vi "Title Font Read.vi"(4 "error in (no error)":errorcluster, 6 "Container State":T14, 7 "Display State In":T1={"Properties"={"Chart"={"ChartName"="Chart", "AntiAliasing"=3, "background"={"Color"={"Color"=0, "alpha"=76}, "HatchStyle"=76, "GradientStyle"=0}}, "ChartArea"={"Background"={"Color"={"Color"=0, "alpha"=76}, "HatchStyle"=76, "GradientStyle"=0}, "Border"={"color"={"Color"=0, "alpha"=76}, "DashStyle"=enum."NotSet", "Width"=2}, "3D"={"Enable 3D"=FALSE, "LightStyle"=enum."Realistic", "PointGapDepth"=150, "PointDepth"=120, "Perspective"=6, "WallWidth"=0}}, "Title"={"Enable"=FALSE, "Title"="My Title", "Docking"=0, "Over Plot?"=FALSE, "Font"={"Name"="Arial", "Size"=16.0, "style"=0, "Color"={"Color"=0, "alpha"=76}}, "Background"={"Color"={"Color"=0, "alpha"=76}, "HatchStyle"=76, "GradientStyle"=11711154}}, "Legend"={"Title"="Legend", "TitleSeparator"=enum."None", "Over Plot?"=FALSE, "Docking"=enum."Top", "Border"={"color"={"Color"=0, "alpha"=76}, "DashStyle"=enum."Solid", "Width"=2}, "Background"={"Color"={"Color"=0, "alpha"=76}, "HatchStyle"=76, "GradientStyle"=0}}, "Series"={"Name"="", "Palette"=enum."Bright", "YAxisType"=enum."Secondary", "XAxisType"=enum."Primary", "ChartType"=0, "Border"={"color"={"Color"=0, "alpha"=76}, "DashStyle"=enum."Solid", "Width"=2}, "Color"={"Color"=0, "alpha"=76}, "Marker"={"MarkerStyle"=enum."Triangle", "Size"=12, "Step"=12, "Color"={"Color"=0, "alpha"=76}}}, "Axes"={"Axis-X"={"Enabled"=0, "Title"="", "LineWidth"=2, "ArrowStyle"=1, "IsMarginVisible"=FALSE, "IsMarksNextToAxis"=FALSE, "IsReversed"=FALSE, "IsStartedFromZero"=FALSE}, "Axis-Y"={"Enabled"=0, "Title"="", "LineWidth"=2, "ArrowStyle"=1, "IsMarginVisible"=FALSE, "IsMarksNextToAxis"=FALSE, "IsReversed"=FALSE, "IsStartedFromZero"=FALSE}, "Axis-X2"={"Enabled"=0, "Title"="", "LineWidth"=2, "ArrowStyle"=1, "IsMarginVisible"=FALSE, "IsMarksNextToAxis"=FALSE, "IsReversed"=FALSE, "IsStartedFromZero"=FALSE}, "Axis-Y2"={"Enabled"=0, "Title"="", "LineWidth"=2, "ArrowStyle"=1, "IsMarginVisible"=FALSE, "IsMarksNextToAxis"=FALSE, "IsReversed"=FALSE, "IsStartedFromZero"=FALSE}}}, ".NET"={"Chart"=refnum}, "Runtime Modification"=FALSE} {"Properties"."Axes"."Axis-Y2"."ArrowStyle" items=["None", "Triangle", "SharpTriangle", "Lines"]; "Properties"."Axes"."Axis-Y2"."Enabled" items=["Auto", "True", "False"]; "Properties"."Axes"."Axis-X2"."ArrowStyle" items=["None", "Triangle", "SharpTriangle", "Lines"]; "Properties"."Axes"."Axis-X2"."Enabled" items=["Auto", "True", "False"]; "Properties"."Axes"."Axis-Y"."ArrowStyle" items=["None", "Triangle", "SharpTriangle", "Lines"]; "Properties"."Axes"."Axis-Y"."Enabled" items=["Auto", "True", "False"]; "Properties"."Axes"."Axis-X"."ArrowStyle" items=["None", "Triangle", "SharpTriangle", "Lines"]; "Properties"."Axes"."Axis-X"."Enabled" items=["Auto", "True", "False"]; "Properties"."Chart"."background"."GradientStyle" items=["None", "LeftRight", "TopBottom", "Center", "DiagonalLeft", "DiagonalRight", "HorizontalCenter", "VerticalCenter"]; "Properties"."Chart"."background"."HatchStyle" items=["None", "BackwardDiagonal", "Cross", "DarkDownwardDiagonal", "DarkHorizontal", "DarkUpwardDiagonal", "DarkVertical", "DashedDownwardDiagonal", "DashedHorizontal", "DashedUpwardDiagonal", "DashedVertical", "DiagonalBrick", "DiagonalCross", "Divot", "DottedDiamond", "DottedGrid", "ForwardDiagonal", "Horizontal", "HorizontalBrick", "LargeCheckerBoard", "LargeConfetti", "LargeGrid", "LightDownwardDiagonal", "LightHorizontal", "LightUpwardDiagonal", "LightVertical", "NarrowHorizontal", "NarrowVertical", "OutlinedDiamond", "Percent05", "Percent10", "Percent20", "Percent25", "Percent30", "Percent40", "Percent50", "Percent60", "Percent70", "Percent75", "Percent80", "Percent90", "Plaid", "Shingle", "SmallCheckerBoard", "SmallConfetti", "SmallGrid", "SolidDiamond", "Sphere", "Trellis", "Vertical", "Wave", "Weave", "WideDownwardDiagonal", "WideUpwardDiagonal", "ZigZag"]; "Properties"."Chart"."background"."Color"."alpha" scale=0.0..255.0; "Properties"."Chart"."AntiAliasing" items=["None", "Text", "Graphics", "All"]; "Properties"."Series"."Marker"."Color"."alpha" scale=0.0..255.0; "Properties"."Series"."Color"."alpha" scale=0.0..255.0; "Properties"."Series"."Border"."color"."alpha" scale=0.0..255.0; "Properties"."Series"."ChartType" items=["Point", "FastPoint", "Bubble", "Line", "Spline", "StepLine", "FastLine", "Bar", "StackedBar", "StackedBar100", "Column", "StackedColumn", "StackedColumn100", "Area", "SplineArea", "StackedArea", "StackedArea100", "Pie", "Doughnut", "Stock", "Candlestick", "Range", "SplineRange", "RangeBar", "RangeColumn", "Radar", "Polar", "ErrorBar", "BoxPlot", "Renko", "ThreeLineBreak", "Kagi", "PointAndFigure", "Funnel", "Pyramid"]; "Properties"."ChartArea"."Border"."color"."alpha" scale=0.0..255.0; "Properties"."ChartArea"."Background"."GradientStyle" items=["None", "LeftRight", "TopBottom", "Center", "DiagonalLeft", "DiagonalRight", "HorizontalCenter", "VerticalCenter"]; "Properties"."ChartArea"."Background"."HatchStyle" items=["None", "BackwardDiagonal", "Cross", "DarkDownwardDiagonal", "DarkHorizontal", "DarkUpwardDiagonal", "DarkVertical", "DashedDownwardDiagonal", "DashedHorizontal", "DashedUpwardDiagonal", "DashedVertical", "DiagonalBrick", "DiagonalCross", "Divot", "DottedDiamond", "DottedGrid", "ForwardDiagonal", "Horizontal", "HorizontalBrick", "LargeCheckerBoard", "LargeConfetti", "LargeGrid", "LightDownwardDiagonal", "LightHorizontal", "LightUpwardDiagonal", "LightVertical", "NarrowHorizontal", "NarrowVertical", "OutlinedDiamond", "Percent05", "Percent10", "Percent20", "Percent25", "Percent30", "Percent40", "Percent50", "Percent60", "Percent70", "Percent75", "Percent80", "Percent90", "Plaid", "Shingle", "SmallCheckerBoard", "SmallConfetti", "SmallGrid", "SolidDiamond", "Sphere", "Trellis", "Vertical", "Wave", "Weave", "WideDownwardDiagonal", "WideUpwardDiagonal", "ZigZag"]; "Properties"."ChartArea"."Background"."Color"."alpha" scale=0.0..255.0; "Properties"."Legend"."Background"."GradientStyle" items=["None", "LeftRight", "TopBottom", "Center", "DiagonalLeft", "DiagonalRight", "HorizontalCenter", "VerticalCenter"]; "Properties"."Legend"."Background"."HatchStyle" items=["None", "BackwardDiagonal", "Cross", "DarkDownwardDiagonal", "DarkHorizontal", "DarkUpwardDiagonal", "DarkVertical", "DashedDownwardDiagonal", "DashedHorizontal", "DashedUpwardDiagonal", "DashedVertical", "DiagonalBrick", "DiagonalCross", "Divot", "DottedDiamond", "DottedGrid", "ForwardDiagonal", "Horizontal", "HorizontalBrick", "LargeCheckerBoard", "LargeConfetti", "LargeGrid", "LightDownwardDiagonal", "LightHorizontal", "LightUpwardDiagonal", "LightVertical", "NarrowHorizontal", "NarrowVertical", "OutlinedDiamond", "Percent05", "Percent10", "Percent20", "Percent25", "Percent30", "Percent40", "Percent50", "Percent60", "Percent70", "Percent75", "Percent80", "Percent90", "Plaid", "Shingle", "SmallCheckerBoard", "SmallConfetti", "SmallGrid", "SolidDiamond", "Sphere", "Trellis", "Vertical", "Wave", "Weave", "WideDownwardDiagonal", "WideUpwardDiagonal", "ZigZag"]; "Properties"."Legend"."Background"."Color"."alpha" scale=0.0..255.0; "Properties"."Legend"."Border"."color"."alpha" scale=0.0..255.0; "Properties"."Title"."Background"."GradientStyle" items=["None", "LeftRight", "TopBottom", "Center", "DiagonalLeft", "DiagonalRight", "HorizontalCenter", "VerticalCenter"]; "Properties"."Title"."Background"."HatchStyle" items=["None", "BackwardDiagonal", "Cross", "DarkDownwardDiagonal", "DarkHorizontal", "DarkUpwardDiagonal", "DarkVertical", "DashedDownwardDiagonal", "DashedHorizontal", "DashedUpwardDiagonal", "DashedVertical", "DiagonalBrick", "DiagonalCross", "Divot", "DottedDiamond", "DottedGrid", "ForwardDiagonal", "Horizontal", "HorizontalBrick", "LargeCheckerBoard", "LargeConfetti", "LargeGrid", "LightDownwardDiagonal", "LightHorizontal", "LightUpwardDiagonal", "LightVertical", "NarrowHorizontal", "NarrowVertical", "OutlinedDiamond", "Percent05", "Percent10", "Percent20", "Percent25", "Percent30", "Percent40", "Percent50", "Percent60", "Percent70", "Percent75", "Percent80", "Percent90", "Plaid", "Shingle", "SmallCheckerBoard", "SmallConfetti", "SmallGrid", "SolidDiamond", "Sphere", "Trellis", "Vertical", "Wave", "Weave", "WideDownwardDiagonal", "WideUpwardDiagonal", "ZigZag"]; "Properties"."Title"."Background"."Color"."alpha" scale=0.0..255.0; "Properties"."Title"."Font"."Color"."alpha" scale=0.0..255.0; "Properties"."Title"."Font"."style" items=["Regular"=0, "Bold"=1, "Italic"=2, "Underline"=4, "Strikeout"=8]; "Properties"."Title"."Font"."Size" min=4.0 max=100.0; "Properties"."Title"."Docking" items=["Top", "Right", "Bottom", "Left", "None"]}) -> (0 "error out":errorcluster, 2 "Value":T9={"Name"="Arial", "Size"=16.0, "style"=0, "Color"={"Color"=0, "alpha"=76}} {"Color"."alpha" scale=0.0..255.0; "style" items=["Regular"=0, "Bold"=1, "Italic"=2, "Underline"=4, "Strikeout"=8]; "Size" min=4.0 max=100.0}, 3 "Display State Out":T1={"Properties"={"Chart"={"ChartName"="Chart", "AntiAliasing"=3, "background"={"Color"={"Color"=0, "alpha"=76}, "HatchStyle"=76, "GradientStyle"=0}}, "ChartArea"={"Background"={"Color"={"Color"=0, "alpha"=76}, "HatchStyle"=76, "GradientStyle"=0}, "Border"={"color"={"Color"=0, "alpha"=76}, "DashStyle"=enum."NotSet", "Width"=2}, "3D"={"Enable 3D"=FALSE, "LightStyle"=enum."Realistic", "PointGapDepth"=150, "PointDepth"=120, "Perspective"=6, "WallWidth"=0}}, "Title"={"Enable"=FALSE, "Title"="My Title", "Docking"=0, "Over Plot?"=FALSE, "Font"={"Name"="Arial", "Size"=16.0, "style"=0, "Color"={"Color"=0, "alpha"=76}}, "Background"={"Color"={"Color"=0, "alpha"=76}, "HatchStyle"=76, "GradientStyle"=11711154}}, "Legend"={"Title"="Legend", "TitleSeparator"=enum."None", "Over Plot?"=FALSE, "Docking"=enum."Top", "Border"={"color"={"Color"=0, "alpha"=76}, "DashStyle"=enum."Solid", "Width"=2}, "Background"={"Color"={"Color"=0, "alpha"=76}, "HatchStyle"=76, "GradientStyle"=0}}, "Series"={"Name"="", "Palette"=enum."Bright", "YAxisType"=enum."Secondary", "XAxisType"=enum."Primary", "ChartType"=0, "Border"={"color"={"Color"=0, "alpha"=76}, "DashStyle"=enum."Solid", "Width"=2}, "Color"={"Color"=0, "alpha"=76}, "Marker"={"MarkerStyle"=enum."Triangle", "Size"=12, "Step"=12, "Color"={"Color"=0, "alpha"=76}}}, "Axes"={"Axis-X"={"Enabled"=0, "Title"="", "LineWidth"=2, "ArrowStyle"=1, "IsMarginVisible"=FALSE, "IsMarksNextToAxis"=FALSE, "IsReversed"=FALSE, "IsStartedFromZero"=FALSE}, "Axis-Y"={"Enabled"=0, "Title"="", "LineWidth"=2, "ArrowStyle"=1, "IsMarginVisible"=FALSE, "IsMarksNextToAxis"=FALSE, "IsReversed"=FALSE, "IsStartedFromZero"=FALSE}, "Axis-X2"={"Enabled"=0, "Title"="", "LineWidth"=2, "ArrowStyle"=1, "IsMarginVisible"=FALSE, "IsMarksNextToAxis"=FALSE, "IsReversed"=FALSE, "IsStartedFromZero"=FALSE}, "Axis-Y2"={"Enabled"=0, "Title"="", "LineWidth"=2, "ArrowStyle"=1, "IsMarginVisible"=FALSE, "IsMarksNextToAxis"=FALSE, "IsReversed"=FALSE, "IsStartedFromZero"=FALSE}}}, ".NET"={"Chart"=refnum}, "Runtime Modification"=FALSE} {"Properties"."Axes"."Axis-Y2"."ArrowStyle" items=["None", "Triangle", "SharpTriangle", "Lines"]; "Properties"."Axes"."Axis-Y2"."Enabled" items=["Auto", "True", "False"]; "Properties"."Axes"."Axis-X2"."ArrowStyle" items=["None", "Triangle", "SharpTriangle", "Lines"]; "Properties"."Axes"."Axis-X2"."Enabled" items=["Auto", "True", "False"]; "Properties"."Axes"."Axis-Y"."ArrowStyle" items=["None", "Triangle", "SharpTriangle", "Lines"]; "Properties"."Axes"."Axis-Y"."Enabled" items=["Auto", "True", "False"]; "Properties"."Axes"."Axis-X"."ArrowStyle" items=["None", "Triangle", "SharpTriangle", "Lines"]; "Properties"."Axes"."Axis-X"."Enabled" items=["Auto", "True", "False"]; "Properties"."Chart"."background"."GradientStyle" items=["None", "LeftRight", "TopBottom", "Center", "DiagonalLeft", "DiagonalRight", "HorizontalCenter", "VerticalCenter"]; "Properties"."Chart"."background"."HatchStyle" items=["None", "BackwardDiagonal", "Cross", "DarkDownwardDiagonal", "DarkHorizontal", "DarkUpwardDiagonal", "DarkVertical", "DashedDownwardDiagonal", "DashedHorizontal", "DashedUpwardDiagonal", "DashedVertical", "DiagonalBrick", "DiagonalCross", "Divot", "DottedDiamond", "DottedGrid", "ForwardDiagonal", "Horizontal", "HorizontalBrick", "LargeCheckerBoard", "LargeConfetti", "LargeGrid", "LightDownwardDiagonal", "LightHorizontal", "LightUpwardDiagonal", "LightVertical", "NarrowHorizontal", "NarrowVertical", "OutlinedDiamond", "Percent05", "Percent10", "Percent20", "Percent25", "Percent30", "Percent40", "Percent50", "Percent60", "Percent70", "Percent75", "Percent80", "Percent90", "Plaid", "Shingle", "SmallCheckerBoard", "SmallConfetti", "SmallGrid", "SolidDiamond", "Sphere", "Trellis", "Vertical", "Wave", "Weave", "WideDownwardDiagonal", "WideUpwardDiagonal", "ZigZag"]; "Properties"."Chart"."background"."Color"."alpha" scale=0.0..255.0; "Properties"."Chart"."AntiAliasing" items=["None", "Text", "Graphics", "All"]; "Properties"."Series"."Marker"."Color"."alpha" scale=0.0..255.0; "Properties"."Series"."Color"."alpha" scale=0.0..255.0; "Properties"."Series"."Border"."color"."alpha" scale=0.0..255.0; "Properties"."Series"."ChartType" items=["Point", "FastPoint", "Bubble", "Line", "Spline", "StepLine", "FastLine", "Bar", "StackedBar", "StackedBar100", "Column", "StackedColumn", "StackedColumn100", "Area", "SplineArea", "StackedArea", "StackedArea100", "Pie", "Doughnut", "Stock", "Candlestick", "Range", "SplineRange", "RangeBar", "RangeColumn", "Radar", "Polar", "ErrorBar", "BoxPlot", "Renko", "ThreeLineBreak", "Kagi", "PointAndFigure", "Funnel", "Pyramid"]; "Properties"."ChartArea"."Border"."color"."alpha" scale=0.0..255.0; "Properties"."ChartArea"."Background"."GradientStyle" items=["None", "LeftRight", "TopBottom", "Center", "DiagonalLeft", "DiagonalRight", "HorizontalCenter", "VerticalCenter"]; "Properties"."ChartArea"."Background"."HatchStyle" items=["None", "BackwardDiagonal", "Cross", "DarkDownwardDiagonal", "DarkHorizontal", "DarkUpwardDiagonal", "DarkVertical", "DashedDownwardDiagonal", "DashedHorizontal", "DashedUpwardDiagonal", "DashedVertical", "DiagonalBrick", "DiagonalCross", "Divot", "DottedDiamond", "DottedGrid", "ForwardDiagonal", "Horizontal", "HorizontalBrick", "LargeCheckerBoard", "LargeConfetti", "LargeGrid", "LightDownwardDiagonal", "LightHorizontal", "LightUpwardDiagonal", "LightVertical", "NarrowHorizontal", "NarrowVertical", "OutlinedDiamond", "Percent05", "Percent10", "Percent20", "Percent25", "Percent30", "Percent40", "Percent50", "Percent60", "Percent70", "Percent75", "Percent80", "Percent90", "Plaid", "Shingle", "SmallCheckerBoard", "SmallConfetti", "SmallGrid", "SolidDiamond", "Sphere", "Trellis", "Vertical", "Wave", "Weave", "WideDownwardDiagonal", "WideUpwardDiagonal", "ZigZag"]; "Properties"."ChartArea"."Background"."Color"."alpha" scale=0.0..255.0; "Properties"."Legend"."Background"."GradientStyle" items=["None", "LeftRight", "TopBottom", "Center", "DiagonalLeft", "DiagonalRight", "HorizontalCenter", "VerticalCenter"]; "Properties"."Legend"."Background"."HatchStyle" items=["None", "BackwardDiagonal", "Cross", "DarkDownwardDiagonal", "DarkHorizontal", "DarkUpwardDiagonal", "DarkVertical", "DashedDownwardDiagonal", "DashedHorizontal", "DashedUpwardDiagonal", "DashedVertical", "DiagonalBrick", "DiagonalCross", "Divot", "DottedDiamond", "DottedGrid", "ForwardDiagonal", "Horizontal", "HorizontalBrick", "LargeCheckerBoard", "LargeConfetti", "LargeGrid", "LightDownwardDiagonal", "LightHorizontal", "LightUpwardDiagonal", "LightVertical", "NarrowHorizontal", "NarrowVertical", "OutlinedDiamond", "Percent05", "Percent10", "Percent20", "Percent25", "Percent30", "Percent40", "Percent50", "Percent60", "Percent70", "Percent75", "Percent80", "Percent90", "Plaid", "Shingle", "SmallCheckerBoard", "SmallConfetti", "SmallGrid", "SolidDiamond", "Sphere", "Trellis", "Vertical", "Wave", "Weave", "WideDownwardDiagonal", "WideUpwardDiagonal", "ZigZag"]; "Properties"."Legend"."Background"."Color"."alpha" scale=0.0..255.0; "Properties"."Legend"."Border"."color"."alpha" scale=0.0..255.0; "Properties"."Title"."Background"."GradientStyle" items=["None", "LeftRight", "TopBottom", "Center", "DiagonalLeft", "DiagonalRight", "HorizontalCenter", "VerticalCenter"]; "Properties"."Title"."Background"."HatchStyle" items=["None", "BackwardDiagonal", "Cross", "DarkDownwardDiagonal", "DarkHorizontal", "DarkUpwardDiagonal", "DarkVertical", "DashedDownwardDiagonal", "DashedHorizontal", "DashedUpwardDiagonal", "DashedVertical", "DiagonalBrick", "DiagonalCross", "Divot", "DottedDiamond", "DottedGrid", "ForwardDiagonal", "Horizontal", "HorizontalBrick", "LargeCheckerBoard", "LargeConfetti", "LargeGrid", "LightDownwardDiagonal", "LightHorizontal", "LightUpwardDiagonal", "LightVertical", "NarrowHorizontal", "NarrowVertical", "OutlinedDiamond", "Percent05", "Percent10", "Percent20", "Percent25", "Percent30", "Percent40", "Percent50", "Percent60", "Percent70", "Percent75", "Percent80", "Percent90", "Plaid", "Shingle", "SmallCheckerBoard", "SmallConfetti", "SmallGrid", "SolidDiamond", "Sphere", "Trellis", "Vertical", "Wave", "Weave", "WideDownwardDiagonal", "WideUpwardDiagonal", "ZigZag"]; "Properties"."Title"."Background"."Color"."alpha" scale=0.0..255.0; "Properties"."Title"."Font"."Color"."alpha" scale=0.0..255.0; "Properties"."Title"."Font"."style" items=["Regular"=0, "Bold"=1, "Italic"=2, "Underline"=4, "Strikeout"=8]; "Properties"."Title"."Font"."Size" min=4.0 max=100.0; "Properties"."Title"."Docking" items=["Top", "Right", "Bottom", "Left", "None"]})   [LabVIEW 2014, in "XMSChart.xctl"]
uses:
  XMSChart.xctl
  <vilib>/_xctls/Container State.ctl
  .net.MSChart/Controls/Font.ctl
  .net.MSChart/Controls/Color.ctl
  Ability/State.ctl
  .net.MSChart/Controls/Chart.ctl
  .net.MSChart/Controls/Background.ctl
  .net.MSChart/Controls/ChartArea.ctl
  .net.MSChart/Controls/Border.ctl
  .net.MSChart/Controls/3D.ctl
  .net.MSChart/Controls/Title.ctl
  .net.MSChart/Controls/Legend.ctl
  .net.MSChart/Controls/Series.ctl
  .net.MSChart/Controls/Marker.ctl
  .net.MSChart/Controls/Axis.ctl
  System.Windows.Forms.DataVisualization
  <vilib>/_xctls/XControlSupport.lvlib
panel:
  # "Replace the Value Indicator below with an Indicator of desired type.\nDo not remove this Indicator or the others from the connector pane. \nDo not change the connector pane pattern.\nThe Value Indicator should always be the second terminal from top on the output side in the connector pane."
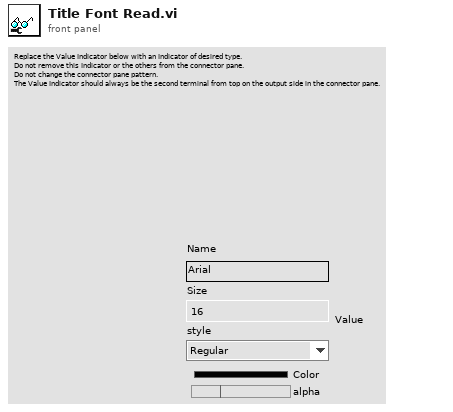
[diagram p1: front panel]
types:
  T1 = typedef "XMSChart.xctl/State.ctl" = cluster{"Properties":cluster{"Chart":T2, "ChartArea":T5, "Title":T8, "Legend":T10, "Series":T11, "Axes":cluster{"Axis-X":T13, "Axis-Y":T13, "Axis-X2":T13, "Axis-Y2":T13}}, ".NET":cluster{"Chart":refnum<k24>}, "Runtime Modification":bool}
  T2 = typedef "XMSChart.xctl/Chart.ctl" = cluster{"ChartName":string, "AntiAliasing":i32, "background":T3}
  T3 = typedef "XMSChart.xctl/Background.ctl" = cluster{"Color":T4, "HatchStyle":i32, "GradientStyle":i32}
  T4 = typedef "XMSChart.xctl/Color.ctl" = cluster{"Color":u32, "alpha":u8}
  T5 = typedef "XMSChart.xctl/ChartArea.ctl" = cluster{"Background":T3, "Border":T6, "3D":T7}
  T6 = typedef "XMSChart.xctl/Border.ctl" = cluster{"color":T4, "DashStyle":enum16{"NotSet", "Dash", "DashDot", "DashDotDot", "Dot", "Solid"}, "Width":i32}
  T7 = typedef "XMSChart.xctl/3D.ctl" = cluster{"Enable 3D":bool, "LightStyle":enum16{"None", "Simplistic", "Realistic"}, "PointGapDepth":i32, "PointDepth":i32, "Perspective":i32, "WallWidth":i32}
  T8 = typedef "XMSChart.xctl/Title.ctl" = cluster{"Enable":bool, "Title":string, "Docking":i32, "Over Plot?":bool, "Font":T9, "Background":T3}
  T9 = typedef "XMSChart.xctl/Font.ctl" = cluster{"Name":string, "Size":dbl, "style":i32, "Color":T4}
  T10 = typedef "XMSChart.xctl/Legend.ctl" = cluster{"Title":string, "TitleSeparator":enum16{"None", "Line", "ThickLine", "DoubleLine", "DashLine", "DotLine", "GradientLine", "ThickGradientLine"}, "Over Plot?":bool, "Docking":enum16{"Top", "Right", "Bottom", "Left", "None"}, "Border":T6, "Background":T3}
  T11 = typedef "XMSChart.xctl/Series.ctl" = cluster{"Name":string, "Palette":enum16{"None", "Bright", "Grayscale", "Excel", "Light", "Pastel", "EarthTones", "SemiTransparent", "Berry", "Chocolate", "Fire", "SeaGreen", "BrightPastel"}, "YAxisType":enum16{"Primary", "Secondary"}, "XAxisType":enum16{"Primary", "Secondary"}, "ChartType":i32, "Border":T6, "Color":T4, "Marker":T12}
  T12 = typedef "XMSChart.xctl/Marker.ctl" = cluster{"MarkerStyle":enum16{"None", "Square", "Circle", "Diamond", "Triangle", "Cross", "Star4", "Star5", "Star6", "Star10"}, "Size":i32, "Step":i32, "Color":T4}
  T13 = typedef "XMSChart.xctl/Axis.ctl" = cluster{"Enabled":i32, "Title":string, "LineWidth":i32, "ArrowStyle":i32, "IsMarginVisible":bool, "IsMarksNextToAxis":bool, "IsReversed":bool, "IsStartedFromZero":bool}
  T14 = typedef "XControlSupport.lvlib/Container State.ctl" = cluster{"Indicator?":bool, "Run Mode?":bool, " Refnum":refnum<vi>}
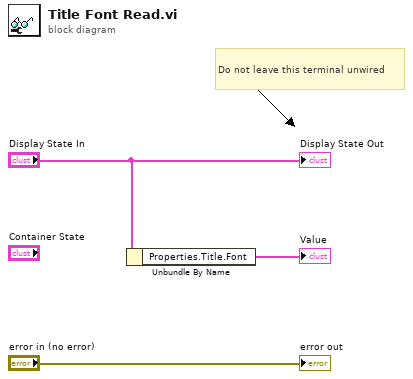
[diagram p0: block diagram]
diagram:
  # "Do not leave this terminal unwired"
  n1 = Unbundle By Name("Display State In") -> ("Properties.Title.Font"=→"Value":T9)
  "error out" <- "error in (no error)"
  "Display State Out" <- "Display State In"
